vi "Turn Left (Jeevan Anga's conflicted copy 2013-04-07).vi"   [LabVIEW 2011]
uses:
  jeevan/Global Variables.vi
types:
  T1 = cluster{"Drive Value Output String":string, "Steer Value Output String":string, "Error Out":errorcluster}
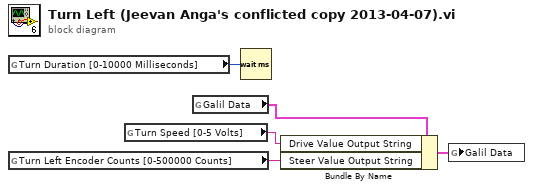
[diagram p0: block diagram]
diagram:
  n1 = global read "Global Variables.vi" "Turn Duration [0-10000 Milliseconds]"() -> (w1:u32)
  n2 = global read "Global Variables.vi" "Turn Left Encoder Counts [0-500000 Counts]"() -> (w2:string)
  n3 = global read "Global Variables.vi" "Turn Speed [0-5 Volts]"() -> (w3:string)
  n4 = global read "Global Variables.vi" "Galil Data"() -> (w4:T1)
  n5 = Wait (ms)(milliseconds to wait=w1) -> ()  [unwired: 1 out]
  n6 = Bundle By Name(cluster=w4, "Drive Value Output String"=w3, "Steer Value Output String"=w2) -> (w5:T1)
  n7 = global write "Global Variables.vi" "Galil Data"(w5) -> ()
